vi "Create Room.vi"(8 "error in (no error)":errorcluster, 10 "Room Name":string, 11 "Room-API in":refnum<class "Room-API.lvclass">) -> (0 "error out":errorcluster, 1 "room_id":string, 2 "created?":bool, 3 "Room-API out":refnum<class "Room-API.lvclass">)   [LabVIEW 2020, in "Room-API.lvclass"]
uses:
  Room-API.lvclass
  Room-API.lvclass/Room-API.ctl
  <vilib>/Utility/error.llb/Error Cluster From Error Code.vi
  <vilib>/ErrorRing/Error Ring.xnode
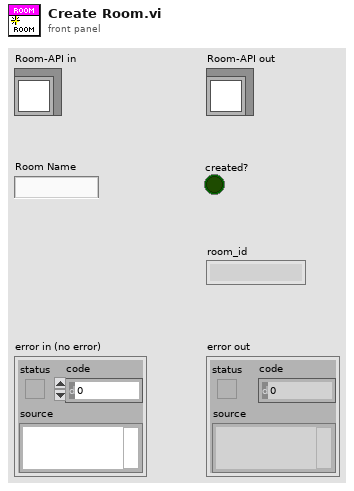
[diagram p1: front panel]
types:
  T1 = typedef "Room-API.lvclass/Single Room.ctl" = cluster{"name":string, "temperature_humidity":string[], "bond":string[], "hue":string[]}
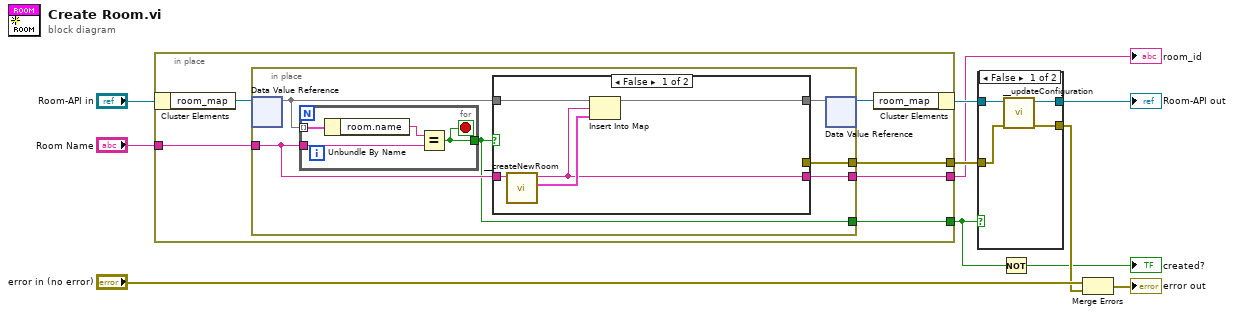
[diagram p0: block diagram]
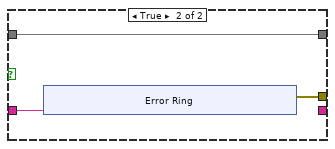
[diagram p3: hidden frame]
diagram:
  n1 = in-place {
    in-place-border: "Room Name" -> [w16]
    in-place-border: [w14] -> w8
    in-place-border: [w13] -> w3
    in-place-border: [w12] -> w1
    n2 = in-place-cluster #1("Room-API in") -> ("room_map"=w17:refnum<data-value>)
    n3 = in-place {
      in-place-border: w16 -> [w22]
      in-place-border: [w20] -> w14
      in-place-border: [w19] -> w13
      in-place-border: [w18] -> w12
      n4 = in-place-dvr #2(w17) -> (w23:map{string, T1})  [unwired: 1 out]
      n5 = for {
        tunnel: w23 -> [w42] mode=indexing
        tunnel: w22 -> [w40]
        tunnel: [w39] -> w19
        stop <- w39 stop-if-true
        n6 = Unbundle By Name(w42) -> ("room.name"=w41:string)
        n7 = Equal?(x=w41, y=w40) -> (x = y?=w39:bool)
      }
      n8 = case shown="False" w19 {
        tunnel: w23 -> [w27 w31]
        tunnel: [w26 w31] -> w21
        tunnel: w22 -> [w28 w30]
        tunnel: [_ w29] -> w20
        tunnel: [w24 _] -> w18
        frame False {
          n9 = call "__createNewRoom.vi"("room_name"=w28) -> ("new_room"=w25:T1, "room_id"=w24:string)  [unwired: 9 in]
          n10 = Insert Into Map(map in=w27, key=w24, value=w25) -> (map out=w26:map{string, T1})  [unwired: 2 out]
        }
        frame True {
          n11 = xnode "Error Ring"("parameter 0"=w30) -> ("error out"=w29:errorcluster)
        }
      }
      n12 = in-place-dvr #2(w21) -> (w15:refnum<data-value>)  [unwired: 1 out]
    }
    n13 = in-place-cluster #1("room_map"=w15) -> (w7:refnum<class "Room-API.lvclass">)
  }
  "room_id" <- w1
  n14 = case shown="False" w3 {
    tunnel: w8 -> [w45 w47]
    tunnel: w7 -> [w46 w48]
    tunnel: [w44 w48] -> w5
    tunnel: [w43 w47] -> w6
    frame False {
      n15 = call "__updateConfiguration.vi"("error in (no error)"=w45, "Room-API in"=w46) -> ("error out"=w43:errorcluster, "Room-API out"=w44:refnum<class "Room-API.lvclass">)  [unwired: 8 in]
    }
    frame True {
    }
  }
  "Room-API out" <- w5
  n16 = Not(x=w3) -> (.not. x?=→"created?":bool)
  n17 = Merge Errors("error in (no error)", w6) -> (→"error out":errorcluster)
